vi "StartStreaming.vi"(8 "error in (no error)":errorcluster, 11 "Camera in":refnum<class "CameraI2COUSB.lvclass">) -> (0 "error out":errorcluster, 3 "Camera out":refnum<class "CameraI2COUSB.lvclass">)   [LabVIEW 2020, in "CameraI2COUSB.lvlib" / "CameraI2COUSB.lvclass"]
doc: "Start streaming"
uses:
  CameraI2COUSB.lvclass
  CameraI2COUSB.lvclass/CameraI2COUSB.ctl
  E:/GitHub/Evaluation_Test/Labview/src/Camera/CameraI2COUSB/Camera/CameraI2COUSB.lvclass
  E:/GitHub/Evaluation_Test/Labview/src/Camera/ICamera/ICamera/ICamera.lvclass
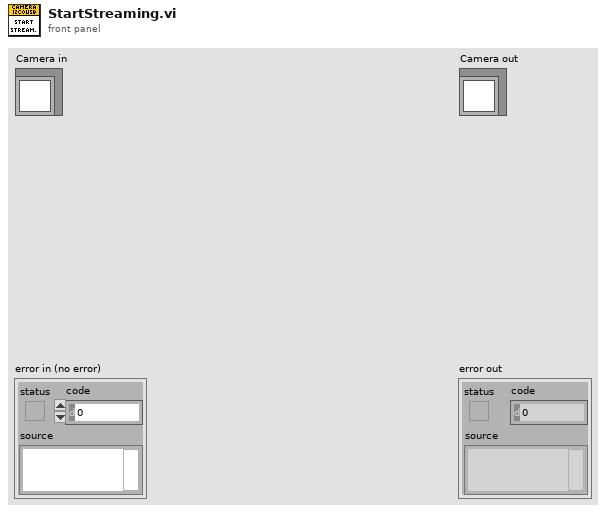
[diagram p1: front panel]
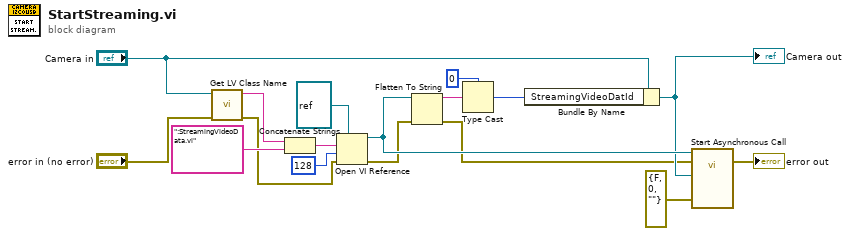
[diagram p0: block diagram]
diagram:
  n1 = call <vilib>:"Get LV Class Name.vi"("error in (no error)"="error in (no error)", "object"="Camera in") -> ("error out"=w3:errorcluster, "class name"=w17:string)  [unwired: 8 in]
  n2 = Concatenate Strings(w17, ":StreamingVideoData.vi" ("string")) -> (w14:string)
  n3 = Open VI Reference(type specifier VI Refnum (for type only)=refnum<vi> refnum, vi path=w14, options=128, error in (no error)=w3) -> (vi reference=w7:refnum<vi>, error out=w2:errorcluster)  [unwired: 2 in]
  n4 = Flatten To String(anything=w7, error in (no error)=w2) -> (data string=w10:string, error out=w1:errorcluster)  [unwired: 2 in, 1 out]
  n5 = Type Cast(type=u32 0, x=w10) -> (*(type *) &x=w8:u32)
  n6 = Bundle By Name(cluster="Camera in", "StreamingVideoDatId"=w8) -> (w4:refnum<class "CameraI2COUSB.lvclass">)
  "Camera out" <- w4
  n7 = call-by-ref "Start Asynchronous Call"(reference=w7, error in=w1, 8:"error in (no error)"=errorcluster {"status"=FALSE, "code"=0, "source"=""} ("error in (no error)"), "CameraDemo in"=w4) -> (error out=→"error out":errorcluster)  [unwired: 8 in, 3 out]
